vi "Main - NaN Value to Zero (SubVI).vi"(11 "Input":sgl) -> (3 "Output":sgl)   [LabVIEW 2019]
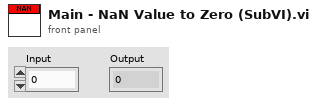
[diagram p1: front panel]
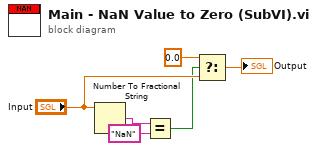
[diagram p0: block diagram]
diagram:
  n1 = Number To Fractional String(number="Input") -> (F-format string=w1:string)  [unwired: 3 in]
  n2 = Equal?(x=w1, y="NaN") -> (x = y?=w3:bool)
  n3 = Select(t=sgl 0.0, s=w3, f="Input") -> (s? t:f=→"Output":sgl)
